vi "pure-cs-scanning.vi"() -> ()   [LabVIEW 2015]
uses:
  raster-scan-params.ctl
  controls/PI-params.ctl
  controls/boolean_info.ctl
  <vilib>/rvi/Emulation/niFpgaGetClockAttributes.vi
  <vilib>/rvi/Emulation/niFpgaSctlEmulationGetInTimedLoop.vi
  <vilib>/rvi/Emulation/niFpgaEmulationReportErrorSimple.vi
  <vilib>/rvi/Emulation/niFpgaProcessEmulError.vi
  <vilib>/rvi/eio/common/nirviEmuTemplateMethod_errors.vi
  <vilib>/rvi/Emulation/niFpgaEmulationIsFPGAContextNoSignature.vi
  <vilib>/rvi/DataTransferAndStorage/Container/Common/niFpgaContainerGetUniqueNameForEmu.vi
  <vilib>/rvi/Memory/Memory_Emulation/niFpgaMemoryEmulationCacheClearOnFirstRun.vi
  <vilib>/rvi/Memory/Memory_Emulation/nirvimemoryEmulationManagerCache_MakeExclusive.vi
  <vilib>/rvi/Memory/Memory_Emulation/niFpgaMemoryEmulationValidateCache.vi
  <vilib>/rvi/Memory/Memory_Emulation/nirvimemoryEmulationManagerCache_InsertValue.vi
  <vilib>/Utility/error.llb/Clear Errors.vi
  <vilib>/rvi/Memory/Memory_Emulation/nirvimemoryEmulationManagerCache_ReleaseExclusive.vi
  <vilib>/rvi/Memory/Memory_Emulation/nirvimemoryEmulationManagerCache_GetValue.vi
  <vilib>/rvi/Memory/Memory_Emulation/nirvimemoryEmulationManagerCache_SetValue.vi
  <vilib>/rvi/DataTransferAndStorage/Container/Common/niFpgaContainerExecOnDevCompGetState.vi
  <vilib>/rvi/Emulation/niFpgaCriticalErrorInLSC.vi
  <vilib>/eio/EIONode/EIONode.xnode
  <vilib>/rvi/DataTransferAndStorage/Container/XNode/niFpgaContainer.xnode
  <vilib>/rvi/DataTransferAndStorage/Register/Emulation/niFpgaRegisterEmulation.vi
  <vilib>/rvi/DataTransferAndStorage/Register/Emulation/niFpgaRegisterEmulationRefIn.vi
  libimaging-cs.lvlib
panel:
  out "case-selected":i16
  out "z-DAC":sgl
  in  "numEntities":i16
  in  "ABORT":bool
  in  "Ki-xy":sgl=0.001 format="%#_13g"
  in  "z-bound":sgl
  in  "xy-bound":sgl
  out "boolean indicators":T1
  out "loggin-fifo-TO":bool=TRUE
  out "input-fifo-TO":bool=TRUE
  in  "raster-scan-params":T2={"TsTicks"=1600, "Stop"=TRUE, "TOL"=0.3, "ramp-rate"=0.0, "z-u-max"=5.0, "PI-params"={"Ki"=0.001, "setpoint"=0.0}} {"z-u-max" format="%#_13g"; "TOL" format="%#_13g"}
  in  "init Z up":sgl
  in  "u_z(0)":sgl format="%#_13g"
  out "ADC-zaxis":fxp<+/-,24,5>
  out "e(0) (threshhold init)":fxp<+/-,16,5>
  out "xref ?":sgl=0.001 format="%#_13g"
  in  "z_UP":sgl=0.001 format="%#_13g"
  in  "zup-N":i16
  out "yref ?":sgl=0.001 format="%#_13g"
  in  "x_ffK":fxp<+/-,16,5>
  in  "trigger-0":bool
  in  "initial case":i16=2
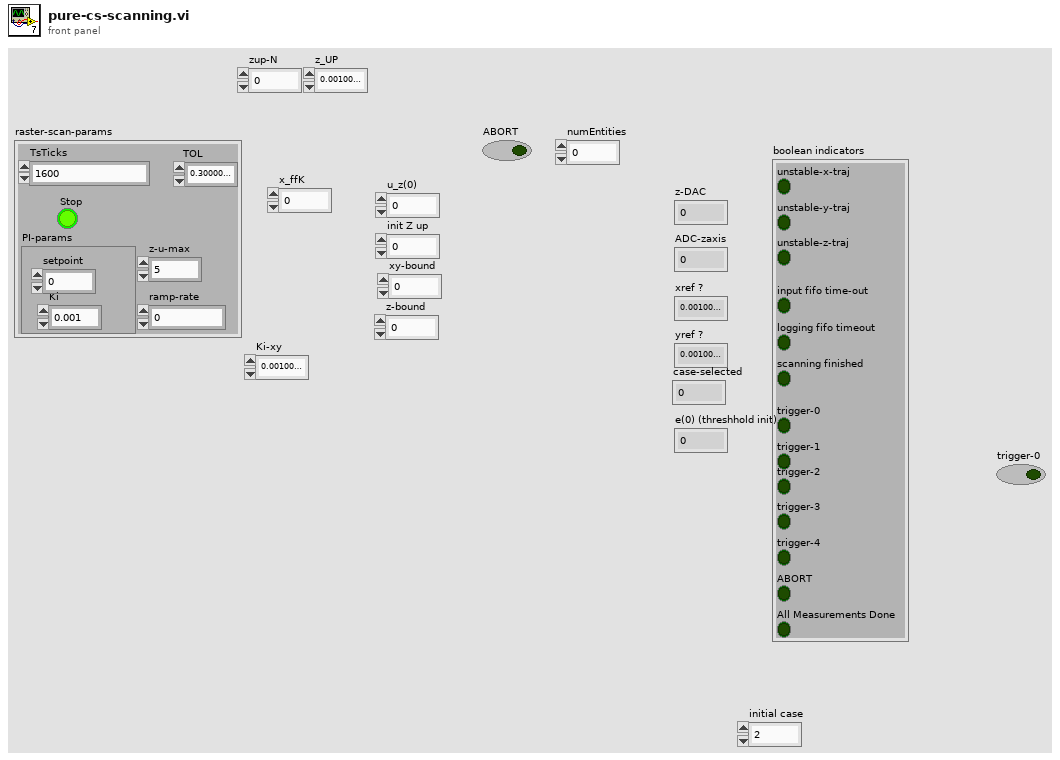
[diagram p1: front panel]
types:
  T1 = typedef "boolean_info.ctl" = cluster{"unstable-z-traj":bool, "input fifo time-out":bool, "logging fifo timeout":bool, "scanning finished":bool, "trigger-1":bool, "trigger-0":bool, "trigger-2":bool, "trigger-3":bool, "trigger-4":bool, "unstable-x-traj":bool, "unstable-y-traj":bool, "ABORT":bool, "All Measurements Done":bool}
  T2 = typedef "raster-scan-params.ctl" = cluster{"TsTicks":u32, "Stop":bool, "TOL":sgl, "ramp-rate":sgl, "z-u-max":sgl, "PI-params":T3}
  T3 = typedef "PI-params.ctl" = cluster{"Ki":sgl, "setpoint":sgl}
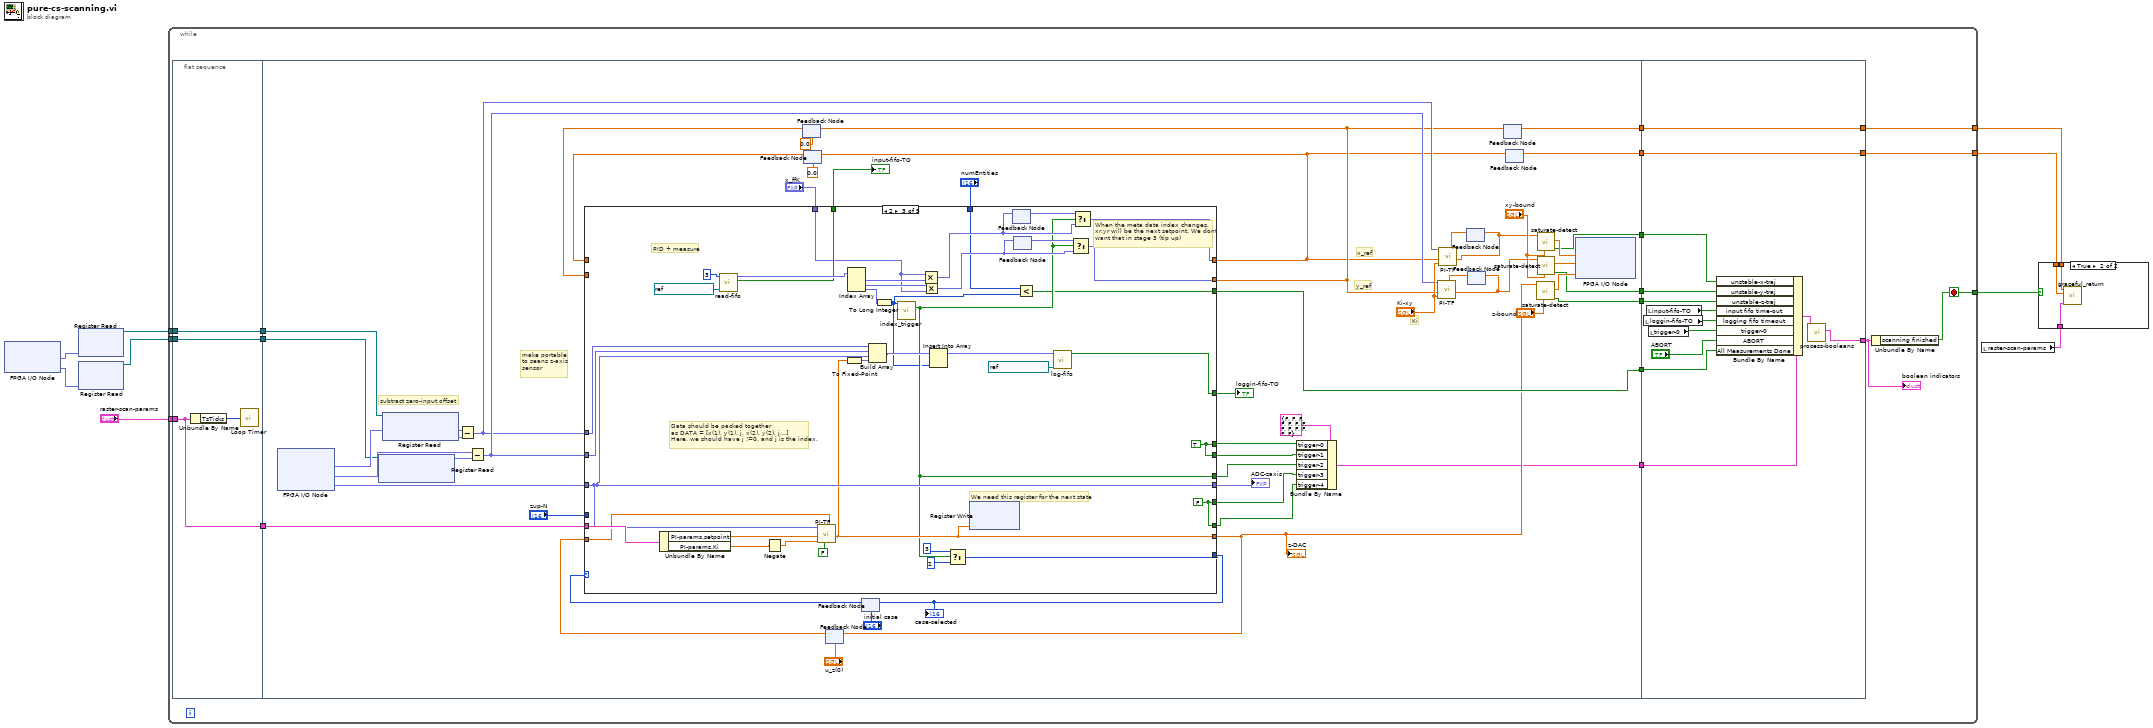
[diagram p0: block diagram]
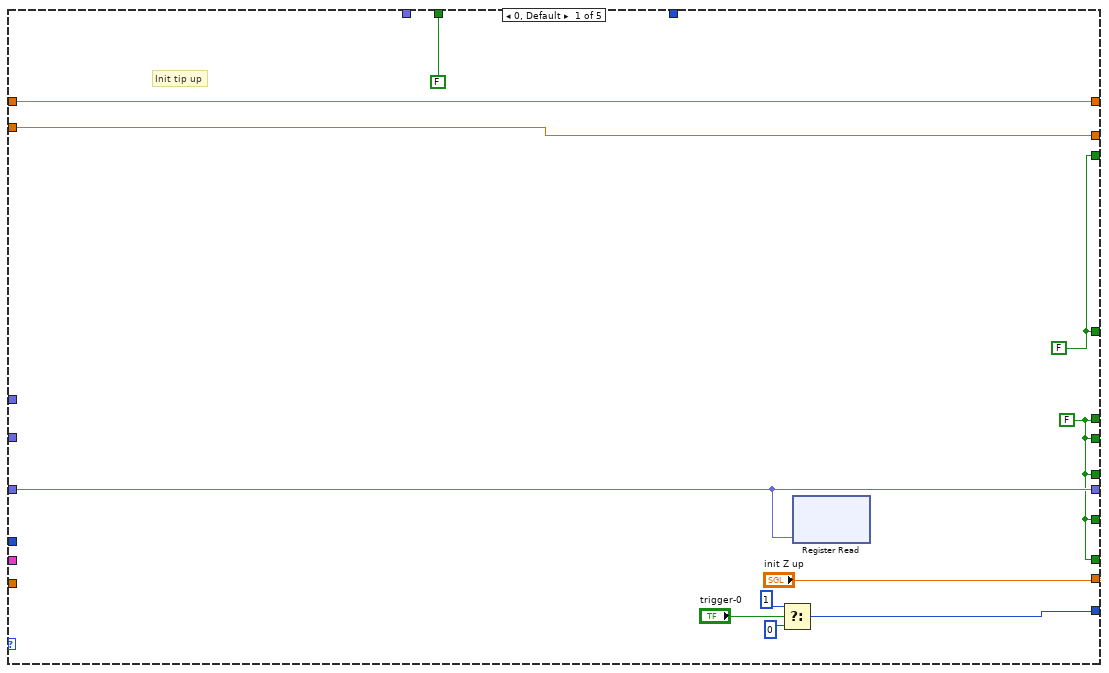
[diagram p3: hidden frame]
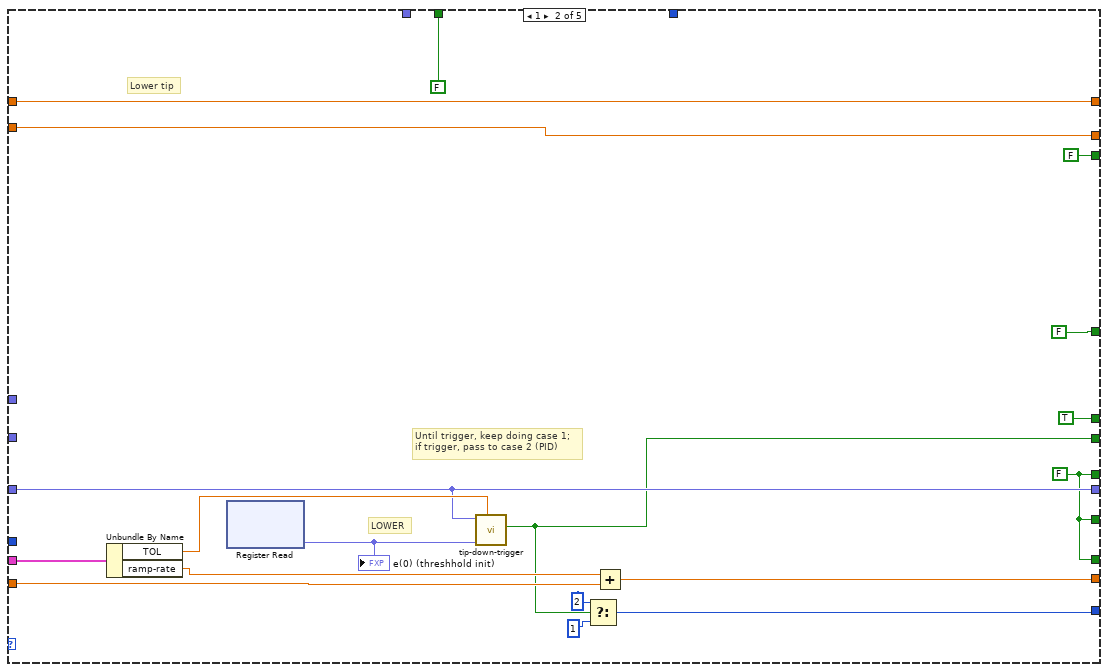
[diagram p4: hidden frame]
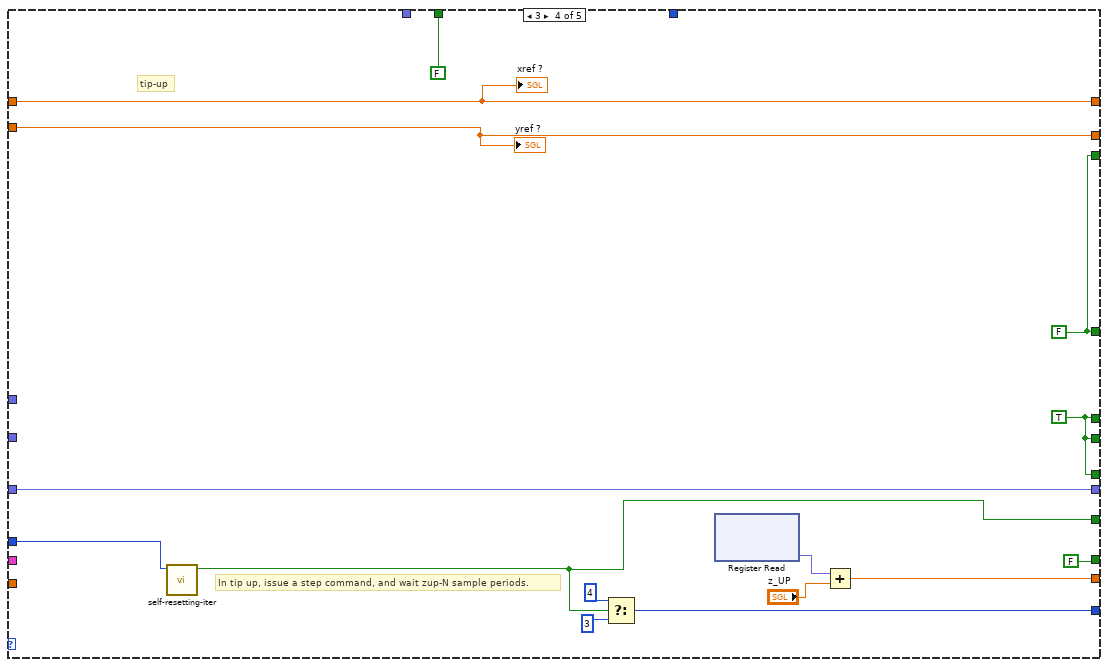
[diagram p5: hidden frame]
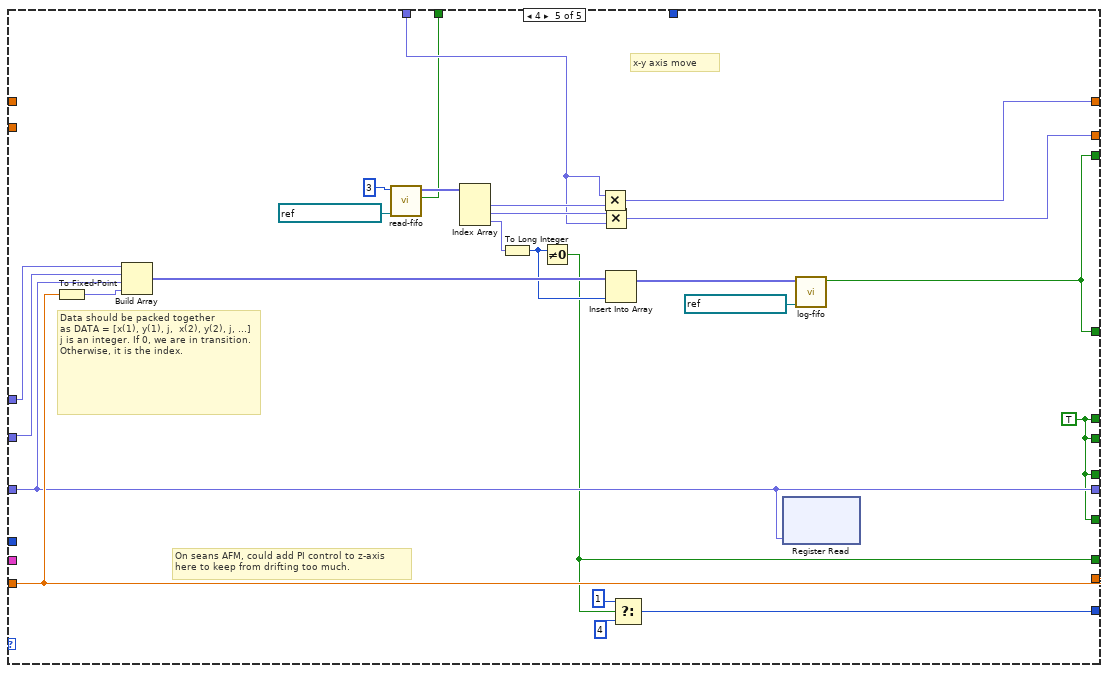
[diagram p6: hidden frame]
diagram:
  n1 = xnode "FPGA I/O Node"() -> ("Mod2/AI0"=w4:fxp<+/-,24,5>, "Mod2/AI1"=w3:fxp<+/-,24,5>)  [unwired: 2 in, 2 out]
  n2 = xnode ("Register Read")("Data"=w3) -> ("Register Out"=w1:refnum<k21>)  [unwired: 1 in]
  n3 = xnode ("Register Read")("Data"=w4) -> ("Register Out"=w2:refnum<k21>)  [unwired: 1 in]
  n4 = while {
    tunnel: "raster-scan-params" -> [w25]
    tunnel: [w24] -> w6
    tunnel: [w23] -> w7
    tunnel: [w20] -> w5
    tunnel: w2 -> [w13]
    tunnel: w1 -> [w11]
    stop <- w20 stop-if-true
    n5 = flat-sequence {
      tunnel: w25 -> [w29]
      tunnel: [w29] -> w26
      tunnel: [w28] -> w14
      tunnel: w13 -> [w28]
      tunnel: [w27] -> w12
      tunnel: w11 -> [w27]
      tunnel: w26 -> [w61]
      tunnel: [w58] -> w22
      tunnel: [w57] -> w21
      tunnel: [w49] -> w18
      tunnel: [w48] -> w17
      tunnel: [w47] -> w16
      tunnel: [w42] -> w15
      tunnel: w14 -> [w41]
      tunnel: w12 -> [w40]
      tunnel: [w32] -> w10
      tunnel: [w200] -> w23
      tunnel: [w201] -> w24
      tunnel: w22 -> [w201]
      tunnel: w21 -> [w200]
      tunnel: [w192] -> w19
      tunnel: w18 -> [w196]
      tunnel: w17 -> [w195]
      tunnel: w16 -> [w194]
      tunnel: w15 -> [w191]
      tunnel: w10 -> [w189]
      frame #0 {
        n6 = Unbundle By Name(w29) -> ("TsTicks"=w30:u32)
        n7 = call "Loop Timer"("Count(Ticks)"=w30) -> ()  [unwired: 1 out]
      }
      frame #1 {
        # "make portable\nto seans z-axis\nsensor"
        # "subtract zero-input offset"
        # "x_ref"
        # "y_ref"
        # "Ki"
        n8 = xnode "FPGA I/O Node"() -> ("Mod2/AI0"=w69:fxp<+/-,24,5>, "Mod2/AI1"=w67:fxp<+/-,24,5>, "Mod2/AI2"=w79:fxp<+/-,24,5>)  [unwired: 3 in, 3 out]
        n9 = xnode ("Register Read")("Register In"=w40) -> ("Data"=w66:fxp<+/-,16,5>)  [unwired: 1 out]
        n10 = xnode ("Register Read")("Register In"=w41) -> ("Data"=w68:fxp<+/-,16,5>)  [unwired: 1 out]
        n11 = Subtract(x=w69, y=w68) -> (x-y=w62:fxp<+/-,25,6>)
        n12 = Subtract(x=w67, y=w66) -> (x-y=w63:fxp<+/-,25,6>)
        n13 = feedback #1(sgl 0.0) -> (w73:sgl)
        n14 = feedback #2(sgl 0.0) -> (w72:sgl)
        n15 = feedback #3("u_z(0)") -> (w71:sgl)
        n16 = feedback #4("initial case") -> (w80:i16)
        n17 = case shown="2" w80 {
          tunnel: [w90 w108 w146 w161 w188] -> w65
          tunnel: w63 -> [_ _ w131 _ w177]
          tunnel: w79 -> [w86 w100 w130 w157 w175]
          tunnel: ["init Z up" w98 w126 w156 w180] -> w39
          tunnel: [w89 w107 w120 w159 w183] -> w59
          tunnel: [w88 w106 w122 w158 w182] -> w60
          tunnel: w73 -> [w88 w106 _ w158 _]
          tunnel: w72 -> [w89 w107 _ w159 _]
          tunnel: w61 -> [_ w102 w139 _ _]
          tunnel: w71 -> [_ w101 w129 _ w180]
          tunnel: [w86 w100 w130 w157 w175] -> w64
          tunnel: w62 -> [_ _ w132 _ w176]
          tunnel: [w84 FALSE w133 w153 w164] -> w46
          tunnel: [FALSE FALSE w136 FALSE w167] -> w45
          tunnel: "x_ffK" -> [_ _ w135 _ w174]
          tunnel: "numEntities" -> [_ _ w116 _ _]
          tunnel: [w84 FALSE w114 w153 w164] -> w42
          tunnel: "zup-N" -> [_ _ _ w152 _]
          tunnel: [w82 w95 w119 w150 w171] -> w35
          tunnel: [w82 w95 w117 w151 w171] -> w34
          tunnel: [w82 w95 w117 FALSE w172] -> w33
          tunnel: [w82 w96 w118 w150 w171] -> w36
          tunnel: [w82 TRUE w118 w150 w171] -> w31
          frame 0, Default {
            w82 = FALSE
            w84 = FALSE
            # "Init tip up"
            n18 = Select(t=i16 1, s="trigger-0", f=i16 0) -> (s? t:f=w90:i16)
            n19 = xnode ("Register Read")("Data"=w86) -> ()  [unwired: 1 in, 1 out]
          }
          frame 1 {
            w95 = FALSE
            # "Until trigger, keep doing case 1;\nif trigger, pass to case 2 (PID)"
            # "LOWER"
            # "Lower tip"
            n20 = Unbundle By Name(w102) -> ("TOL"=w104:sgl, "ramp-rate"=w103:sgl)
            n21 = xnode ("Register Read")() -> ("Data"=w105:fxp<+/-,16,5>)  [unwired: 1 in, 1 out]
            "e(0) (threshhold init)" <- w105
            n22 = call "tip-down-trigger.vi"("TOL"=w104, "Vo"=w105, "e(k)"=w100) -> ("trigger"=w96:bool)  [unwired: 8 in]
            n23 = Select(t=i16 2, s=w96, f=i16 1) -> (s? t:f=w108:i16)
            n24 = Add(x=w103, y=w101) -> (x+y=w98:sgl)
          }
          frame 2 {
            w117 = FALSE
            w118 = TRUE
            # "When the meta data index changes,\nxr,yr will be the next setpoint. We dont\nwant that in stage 3 (tip up)"
            # "We need this register for the next state"
            # "Data should be packed together\nas DATA = [x(1), y(1), j, x(2), y(2), j...]\nHere, we should have j !=0, and j is the index."
            # "PID + measure"
            n25 = Unbundle By Name(w139) -> ("PI-params.setpoint"=w140:sgl, "PI-params.Ki"=w137:sgl)
            n26 = call "read-fifo.vi"("FIFO In"=refnum<k21> "Host_to_FPGA", "numChan"=3) -> ("timout?"=w136:bool, "unpacked-data"=w143:fxp<+/-,16,5>[])  [unwired: 8 in]
            n27 = Negate(x=w137) -> (-x=w138:sgl)
            n28 = call "PI-TF.vi"("u(k-1)"=w129, "reset"=FALSE, "Ki"=w138, "setpoint"=w140, "y(k)"=w130) -> ("u(k)"=w126:sgl)  [unwired: 6 in]
            n29 = To Fixed-Point(number=w126) -> (fixed-point=w128:fxp<+/-,16,5>)  [unwired: 1 in]
            n30 = Index Array(array=w143) -> (element #1=w145:fxp<+/-,16,5>, element #2=w144:fxp<+/-,16,5>, element #3=w142:fxp<+/-,16,5>)  [unwired: 3 in]
            n31 = Build Array(w132, w131, w130, w128) -> (w127:fxp<+/-,25,6>[])
            n32 = To Long Integer(number=w142) -> (32bit integer=w115:i32)
            n33 = call "index_trigger.vi"("fifo-counter"=w115) -> ("index trigger"=w119:bool)  [unwired: 10 in]
            n34 = Multiply(x=w135, y=w145) -> (x*y=w124:fxp<+/-,32,10>)
            n35 = Multiply(x=w144, y=w135) -> (x*y=w121:fxp<+/-,32,10>)
            n36 = Insert Into Array(array=w127, new element=w115) -> (w134:fxp<+/-,25,6>[])  [unwired: 1 in]
            n37 = Select(t=i16 3, s=w119, f=i16 2) -> (s? t:f=w146:i16)
            n38 = xnode ("Register Write")("Data"=w126) -> ()  [unwired: 1 in, 1 out]
            n39 = feedback-in #5(w124) -> ()
            n40 = feedback #5() -> (w125:fxp<+/-,32,10>)  [unwired: 1 in]
            n41 = feedback #6() -> (w123:fxp<+/-,32,10>)  [unwired: 1 in]
            n42 = feedback-in #6(w121) -> ()
            n43 = Less?(x=w116, y=w115) -> (x < y?=w114:bool)
            n44 = call "log-fifo.vi"("FIFO In"=refnum<k21> "fpga-to-host2", "input-data"=w134) -> ("logging-timeout?"=w133:bool)  [unwired: 9 in]
            n45 = Select(t=w123, s=w119, f=w121) -> (s? t:f=w122:fxp<+/-,32,10>)
            n46 = Select(t=w125, s=w119, f=w124) -> (s? t:f=w120:fxp<+/-,32,10>)
          }
          frame 3 {
            w150 = TRUE
            w153 = FALSE
            # "In tip up, issue a step command, and wait zup-N sample periods."
            # "tip-up"
            n47 = call "self-resetting-iter.vi"("zup-N"=w152) -> ("Boolean"=w151:bool)  [unwired: 9 in, 1 out]
            n48 = Select(t=i16 4, s=w151, f=i16 3) -> (s? t:f=w161:i16)
            n49 = xnode ("Register Read")() -> ("Data"=w154:fxp<+/-,16,5>)  [unwired: 1 in, 1 out]
            n50 = Add(x=w154, y="z_UP") -> (x+y=w156:sgl)
            "yref ?" <- w158
            "xref ?" <- w159
          }
          frame 4 {
            w171 = TRUE
            # "On seans AFM, could add PI control to z-axis\nhere to keep from drifting too much."
            # "Data should be packed together\nas DATA = [x(1), y(1), j,  x(2), y(2), j, ...]\nj is an integer. If 0, we are in transition. Otherwise, it is the index."
            # "x-y axis move"
            n51 = To Fixed-Point(number=w180) -> (fixed-point=w173:fxp<+/-,16,5>)  [unwired: 1 in]
            n52 = Build Array(w176, w177, w175, w173) -> (w179:fxp<+/-,25,6>[])
            n53 = call "read-fifo.vi"("FIFO In"=refnum<k21> "Host_to_FPGA", "numChan"=3) -> ("timout?"=w167:bool, "unpacked-data"=w168:fxp<+/-,16,5>[])  [unwired: 8 in]
            n54 = Index Array(array=w168) -> (element #1=w185:fxp<+/-,16,5>, element #2=w184:fxp<+/-,16,5>, element #3=w181:fxp<+/-,16,5>)  [unwired: 3 in]
            n55 = To Long Integer(number=w181) -> (32bit integer=w178:i32)
            n56 = Not Equal To 0?(x=w178) -> (x != 0?=w172:bool)
            n57 = Multiply(x=w174, y=w185) -> (x*y=w183:fxp<+/-,32,10>)
            n58 = Multiply(x=w184, y=w174) -> (x*y=w182:fxp<+/-,32,10>)
            n59 = Insert Into Array(array=w179, new element=w178) -> (w166:fxp<+/-,25,6>[])  [unwired: 1 in]
            n60 = Select(t=i16 1, s=w172, f=i16 4) -> (s? t:f=w188:i16)
            n61 = xnode ("Register Read")("Data"=w175) -> ()  [unwired: 1 in, 1 out]
            n62 = call "log-fifo.vi"("FIFO In"=refnum<k21> "fpga-to-host2", "input-data"=w166) -> ("logging-timeout?"=w164:bool)  [unwired: 9 in]
          }
        }
        "ADC-zaxis" <- w64
        "loggin-fifo-TO" <- w46
        "input-fifo-TO" <- w45
        "z-DAC" <- w39
        "case-selected" <- w65
        n63 = feedback-in #1(w60) -> ()
        n64 = feedback-in #2(w59) -> ()
        n65 = feedback-in #3(w39) -> ()
        n66 = feedback-in #4(w65) -> ()
        n67 = Bundle By Name(cluster=T1 {"unstable-z-traj"=FALSE, "input fifo time-out"=FALSE, "logging fifo timeout"=FALSE, "scanning finished"=FALSE, "trigger-1"=FALSE, "trigger-0"=FALSE, "trigger-2"=FALSE, "trigger-3"=FALSE, "trigger-4"=FALSE, "unstable-x-traj"=FALSE, "unstable-y-traj"=FALSE, "ABORT"=FALSE, "All Measurements Done"=FALSE} ("boolean errors"), "trigger-0"=w31, "trigger-1"=w36, "trigger-2"=w35, "trigger-3"=w34, "trigger-4"=w33) -> (w32:T1)
        n68 = feedback #7() -> (w77:sgl)  [unwired: 1 in]
        n69 = call "PI-TF.vi"("u(k-1)"=w77, "Ki"="Ki-xy", "setpoint"=w59, "y(k)"=w62) -> ("u(k)"=w52:sgl)  [unwired: 7 in]
        n70 = feedback-in #7(w52) -> ()
        n71 = feedback #8() -> (w76:sgl)  [unwired: 1 in]
        n72 = call "PI-TF.vi"("u(k-1)"=w76, "Ki"="Ki-xy", "setpoint"=w60, "y(k)"=w63) -> ("u(k)"=w53:sgl)  [unwired: 7 in]
        n73 = feedback-in #8(w53) -> ()
        n74 = feedback #9() -> (w57:sgl)  [unwired: 1 in]
        n75 = feedback-in #9(w60) -> ()
        n76 = feedback #10() -> (w58:sgl)  [unwired: 1 in]
        n77 = feedback-in #10(w59) -> ()
        n78 = call "saturate-detect.vi"("bound"="z-bound", "x"=w39) -> ("saturated"=w47:bool, "sat(x)"=w51:sgl)  [unwired: 8 in]
        n79 = call "saturate-detect.vi"("bound"="xy-bound", "x"=w52) -> ("saturated"=w49:bool, "sat(x)"=w54:sgl)  [unwired: 8 in]
        n80 = call "saturate-detect.vi"("bound"="xy-bound", "x"=w53) -> ("saturated"=w48:bool, "sat(x)"=w55:sgl)  [unwired: 8 in]
        n81 = xnode "FPGA I/O Node"("Mod1/AO0"=w54, "Mod1/AO1"=w55, "Mod1/AO2"=w51) -> ()  [unwired: 3 in, 3 out]
      }
      frame #2 {
        n82 = local read "loggin-fifo-TO"() -> (w198:bool)
        n83 = local read "input-fifo-TO"() -> (w199:bool)
        n84 = local read "trigger-0"() -> (w197:bool)
        n85 = Bundle By Name(cluster=w189, "unstable-x-traj"=w196, "unstable-y-traj"=w195, "unstable-z-traj"=w194, "input fifo time-out"=w199, "logging fifo timeout"=w198, "trigger-0"=w197, "ABORT"="ABORT", "All Measurements Done"=w191) -> (w190:T1)
        n86 = call "process-booleans.vi"("boolean indicators 2"=w190) -> ("boolean indicators"=w192:T1)  [unwired: 10 in]
      }
    }
    n87 = Unbundle By Name(w19) -> ("scanning finished"=w20:bool)
    "boolean indicators" <- w19
  }
  n88 = local read "raster-scan-params"() -> (w8:T2)
  n89 = case shown="True" w5 {
    tunnel: w7 -> [_ w204]
    tunnel: w6 -> [_ w203]
    tunnel: w8 -> [_ w202]
    frame False {
    }
    frame True {
      n90 = call "graceful_return.vi"("raster-scan-params"=w202, "uy(0)"=w203, "ux(0)"=w204) -> ()  [unwired: 9 in]
    }
  }
